vi "trace_toLVBuffer.vi"(0 "reference in":refnum<class "OSA.lvclass">, 2 "idx latest":bool, 3 "dataType":T1, 4 "trace idx":u32, 5 "error in (no error)":errorcluster) -> (14 "reference out":refnum<class "OSA.lvclass">, 17 "trace length":u32, 19 "error out":errorcluster)   [LabVIEW 2010, in "OSA.lvclass"]
doc: "Reads data from trace buffer and updates labview buffer, access labview buffer with buffer_get.vi \n\nSee buffer_get.vi for X and Y units and formats.\n\nTrace index will be selected either according to the trace idx control or to the trace that most recently received data from an acquisition, (asAcq_dataWaitGet_trace.vi, dataAcq_get_spectrum_trace.vi, dataAcq_get_interferogram_trace.vi). The latter will be selected if idx latest = TRUE."
uses:
  OSA.lvclass
  typeDef/acq_dataType.ctl
  OSA20X_misc.lvlib
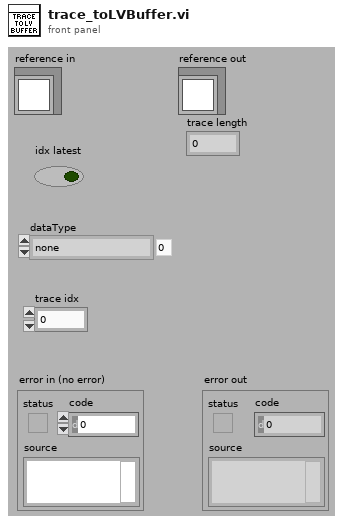
[diagram p1: front panel]
types:
  T1 = typedef "OSA.lvclass/acq_dataType.ctl" = enum16{"none", "interferogram", "spectrum"}
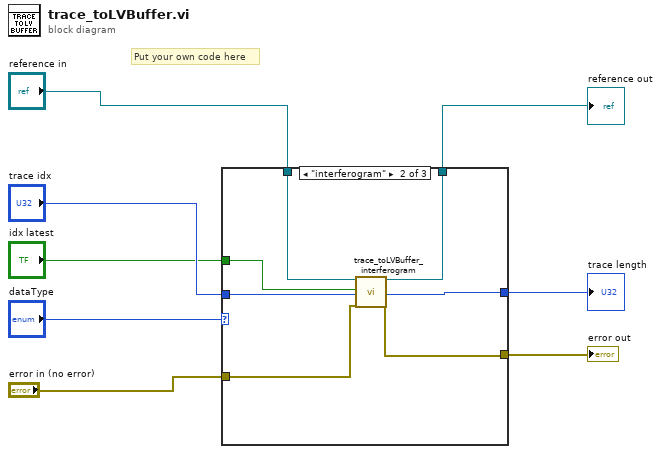
[diagram p0: block diagram]
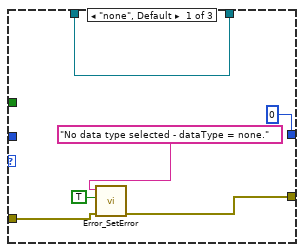
[diagram p2: hidden frame]
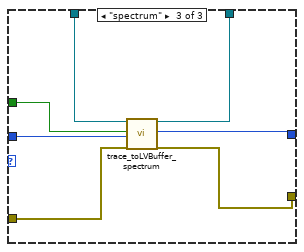
[diagram p3: hidden frame]
diagram:
  # "Put your own code here"
  n1 = case shown="\"interferogram\"" "dataType" {
    tunnel: "reference in" -> [w9 w21 w28]
    tunnel: [w9 w20 w27] -> w3
    tunnel: "error in (no error)" -> [w12 w19 w23]
    tunnel: [w11 w18 w22] -> w8
    tunnel: "idx latest" -> [_ w17 w25]
    tunnel: "trace idx" -> [_ w16 w24]
    tunnel: [u32 0 ("trace length") w15 w26] -> w1
    frame "none", Default {
      n2 = call "Error_SetError.vi"("error in"=w12, "status (true)"=TRUE, "source(\"\")"="No data type selected - dataType = none." ("source(\"\")")) -> ("error out"=w11:errorcluster)  [unwired: 4 in]
    }
    frame "interferogram" {
      n3 = call "trace_toLVBuffer_interferogram.vi"("reference"=w21, "idx latest"=w17, "trace idx interferogram"=w16, "error in (no error)"=w19) -> ("duplicate reference"=w20:refnum<class "OSA.lvclass">, "trace length"=w15:u32, "error out"=w18:errorcluster)  [unwired: 13 in]
    }
    frame "spectrum" {
      n4 = call "trace_toLVBuffer_spectrum.vi"("reference"=w28, "idx latest"=w25, "trace idx spectrum"=w24, "error in (no error)"=w23) -> ("duplicate reference"=w27:refnum<class "OSA.lvclass">, "trace length"=w26:u32, "error out"=w22:errorcluster)  [unwired: 13 in]
    }
  }
  "error out" <- w8
  "reference out" <- w3
  "trace length" <- w1
